vi "SIZE.vi"(8 "error in (no error)":errorcluster, 10 "Remote FileName":string, 11 "FTP in":refnum<class "FTP.lvclass">) -> (0 "error out":errorcluster, 2 "FileSize":i64, 3 "FTP out":refnum<class "FTP.lvclass">)   [LabVIEW 2020, in "FTP.lvlib" / "FTP.lvclass"]
uses:
  FTP.lvclass
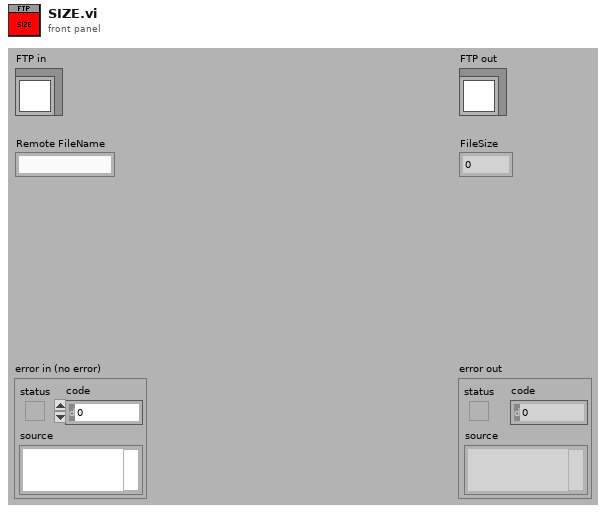
[diagram p1: front panel]
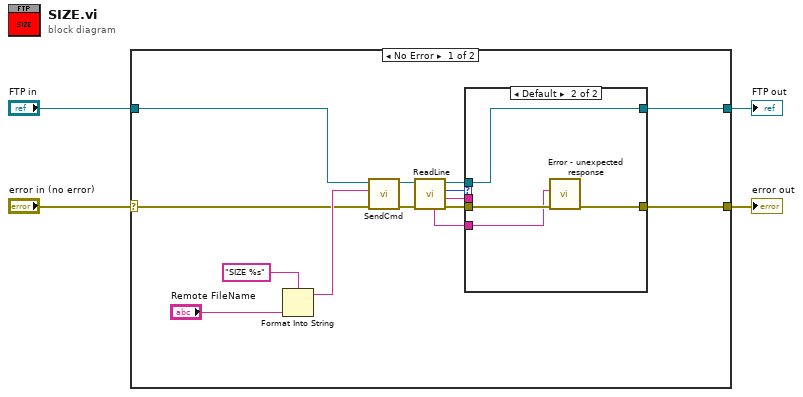
[diagram p0: block diagram]
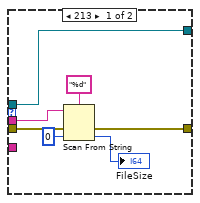
[diagram p2: hidden frame]
diagram:
  n1 = case shown="No Error" "error in (no error)" {
    selector: "error in (no error)" -> [w14 w31]
    tunnel: [w8 w31] -> w3
    tunnel: [w7 w30] -> w1
    tunnel: "FTP in" -> [w15 w30]
    frame No Error {
      n2 = Format Into String(format string="SIZE %s" ("cmd"), "Remote FileName") -> (resulting string=w16:string)  [unwired: 2 in, 1 out]
      n3 = call "SendCmd.vi"("error in (no error)"=w14, "cmd"=w16, "FTP in"=w15) -> ("error out"=w13:errorcluster, "FTP out"=w12:refnum<class "FTP.lvclass">)  [unwired: 7 in]
      n4 = call "ReadLine.vi"("error in (no error)"=w13, "FTP in"=w12) -> ("error out"=w9:errorcluster, "Line"=w6:string, "code"=w10:i32, "FTP out"=w11:refnum<class "FTP.lvclass">, "Full Line"=w5:string)  [unwired: 5 in]
      n5 = case shown="Default" w10 {
        tunnel: w11 -> [w25 w29]
        tunnel: w9 -> [w24 w28]
        tunnel: [w23 w27] -> w8
        tunnel: [w25 w29] -> w7
        tunnel: w6 -> [w22 _]
        tunnel: w5 -> [_ w26]
        frame 213 {
          n6 = Scan From String(format string="%d", input string=w22, error in=w24, default 1=i64 0 ("default value 1")) -> (error out=w23:errorcluster, output 1=→"FileSize":i64)  [unwired: 1 in, 2 out]
        }
        frame Default {
          n7 = call "Error - unexpected response.vi"("error in (no error)"=w28, "Full Response"=w26) -> ("error out"=w27:errorcluster)  [unwired: 9 in]
        }
      }
    }
    frame Error {
    }
  }
  "error out" <- w3
  "FTP out" <- w1
